vi "Write Group Name.vi"(8 "error in (no error)":errorcluster, 10 "Group Name":string, 11 "Write Group Name Msg in":refnum<class "Write Group Name Msg.lvclass">) -> (0 "error out":errorcluster, 3 "Write Group Name Msg out":refnum<class "Write Group Name Msg.lvclass">)   [LabVIEW 2015, in "Write Group Name Msg.lvclass"]
uses:
  Write Group Name Msg.lvclass
  Write Group Name Msg.lvclass/Write Group Name Msg.ctl
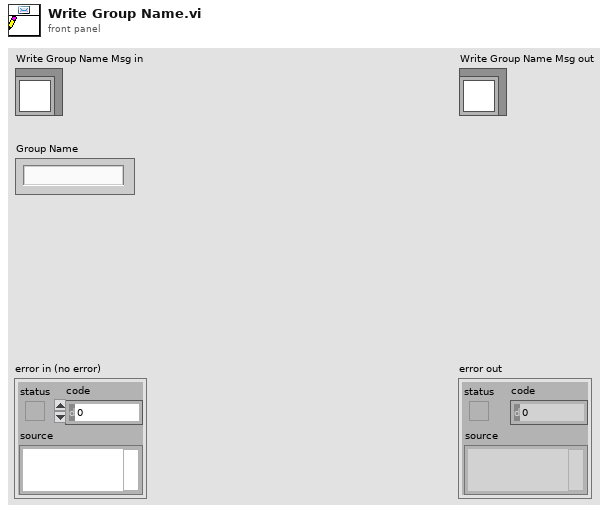
[diagram p1: front panel]
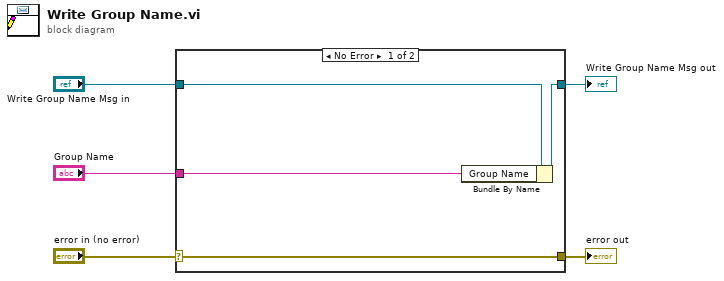
[diagram p0: block diagram]
diagram:
  n1 = case shown="No Error" "error in (no error)" {
    selector: "error in (no error)" -> [w9 w10]
    tunnel: [w9 w10] -> w4
    tunnel: [w7 w11] -> w2
    tunnel: "Write Group Name Msg in" -> [w8 w11]
    tunnel: "Group Name" -> [w6 _]
    frame No Error {
      n2 = Bundle By Name(cluster=w8, "Group Name"=w6) -> (w7:refnum<class "Write Group Name Msg.lvclass">)
    }
    frame Error {
    }
  }
  "error out" <- w4
  "Write Group Name Msg out" <- w2
